vi "ex_4_9.vi"() -> ()   [LabVIEW 2020]
panel:
  out "Numeric":i32
  in  "String":string
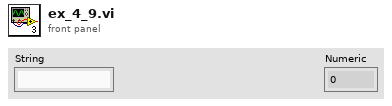
[diagram p1: front panel]
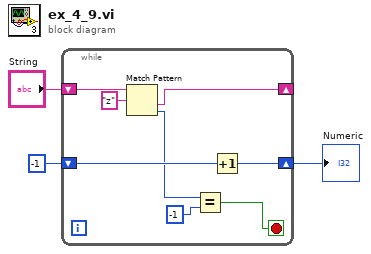
[diagram p0: block diagram]
diagram:
  n1 = while {
    shift-right: [w4] -> _
    shift-left: "String" -> [w11]
    shift-right: [w5] -> w1
    shift-left: -1 -> [w9]
    stop <- w6 stop-if-true
    n2 = Match Pattern(string=w11, regular expression="z" ("search string/char (-)")) -> (after substring=w4:string, offset past match=w8:i32)  [unwired: 1 in, 2 out]
    n3 = Equal?(x=w8, y=-1) -> (x = y?=w6:bool)
    n4 = Increment(x=w9) -> (x+1=w5:i32)
  }
  "Numeric" <- w1
